vi "Handle Error.vi"(8 "error in (no error)":errorcluster, 10 "delimited string":string, 11 "LV Argument Parser in":refnum<class "LV Argument Parser.lvclass">) -> (0 "error out":errorcluster, 2 "Output":string, 3 "LV Argument Parser out":refnum<class "LV Argument Parser.lvclass">)   [LabVIEW 2023, in "LV ArgParse.lvlib" / "LV Argument Parser.lvclass"]
uses:
  LV Argument Parser.lvclass
  LV Argument Parser.lvclass/LV Argument Parser.ctl
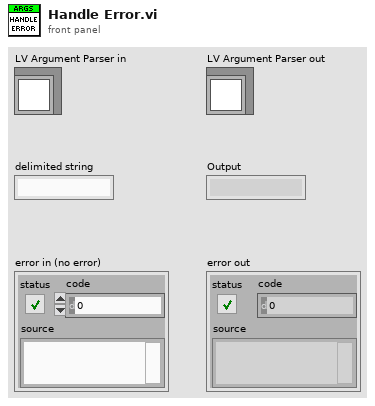
[diagram p1: front panel]
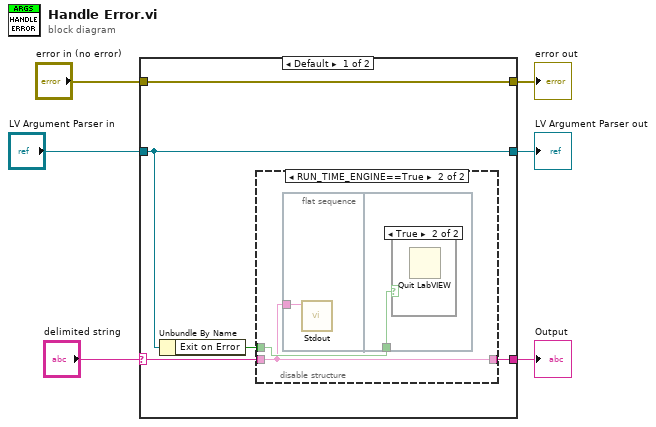
[diagram p0: block diagram]
diagram:
  n1 = case shown="Default" "delimited string" {
    selector: "delimited string" -> [w11 _]
    tunnel: "LV Argument Parser in" -> [w8 w18]
    tunnel: [w8 w18] -> w4
    tunnel: [w10 w17] -> w5
    tunnel: "error in (no error)" -> [w10 w17]
    tunnel: [w9 _] -> w1
    frame Default {
      n2 = Unbundle By Name(w8) -> ("Exit on Error"=w7:bool)
      n3 = disable-structure shown="RUN_TIME_ENGINE==True" {
        disable-tunnel: w11 -> [w12 w13]
        disable-tunnel: [w12 w13] -> w9
        disable-tunnel: w7 -> [_ w14]
        frame condition #0 (active) {
        }
        frame condition #1 {
          n4 = flat-sequence {
            tunnel: w13 -> [w15]
            tunnel: w14 -> [w16]
            frame #0 {
              n5 = call "Stdout.vi"("text"=w15) -> ()  [unwired: 10 in, 1 out]
            }
            frame #1 {
              n6 = case shown="True" w16 {
                frame False {
                }
                frame True {
                  n7 = Quit LabVIEW() -> ()  [unwired: 1 in]
                }
              }
            }
          }
        }
      }
    }
    frame "" {
    }
  }
  "error out" <- w5
  "LV Argument Parser out" <- w4
  "Output" <- w1
